vi "quantizzatore_bipolare.vi"(8 "Segnale input":waveform(dbl), 9 "B (# Bits)":dbl, 10 "Vfs":dbl) -> (0 "Livelli":dbl[](array[numeric]), 1 "Segnale quantizzato":waveform(dbl), 2 "2^B":dbl, 3 "Q":dbl)   [LabVIEW 2009]
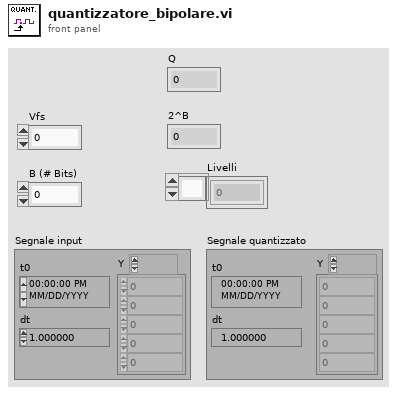
[diagram p1: front panel]
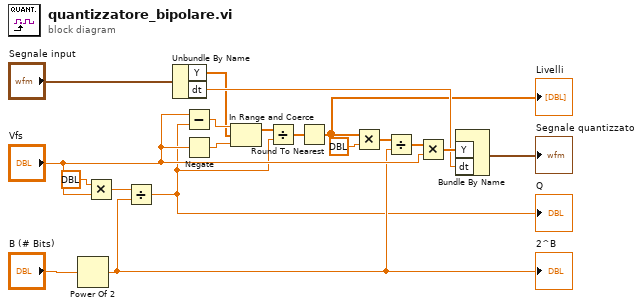
[diagram p0: block diagram]
diagram:
  n1 = Power Of 2(x="B (# Bits)") -> (2^x=w15:dbl)
  "2^B" <- w15
  n2 = Multiply(x=dbl ?, y="Vfs") -> (x*y=w18:dbl)
  n3 = Divide(x=w18, y=w15) -> (x/y=w1:dbl)
  "Q" <- w1
  n4 = Unbundle By Name("Segnale input") -> ("Y"=w5:dbl[], "dt"=w12:dbl)
  n5 = Subtract(x="Vfs", y=w1) -> (x-y=w9:dbl)
  n6 = Negate(x="Vfs") -> (-x=w6:dbl)
  n7 = In Range and Coerce(upper limit=w9, x=w5, lower limit=w6) -> (coerced(x)=w7:dbl[])  [unwired: 1 out]
  n8 = Divide(x=w7, y=w1) -> (x/y=w8:dbl[])
  n9 = Round To Nearest(number=w8) -> (nearest integer value=w4:dbl[])
  "Livelli" <- w4
  n10 = Multiply(x=w4, y=dbl ?) -> (x*y=w2:dbl[])
  n11 = Divide(x=w2, y=w15) -> (x/y=w19:dbl[])
  n12 = Multiply(x=w19, y="Vfs") -> (x*y=w13:dbl[])
  n13 = Bundle By Name("Y"=w13, "dt"=w12) -> (→"Segnale quantizzato":waveform(dbl))  [unwired: 1 in]
